vi "EXAMPLE_REQUEST.vi"() -> ()   [LabVIEW 2016]
uses:
  Response/Response.lvclass
panel:
  in  "Request":T1(ring)=enum."PATCH"
  out "Response Headers":string
  out "Status Description":string
  out "Status Code":dbl
  out "Response Body":string
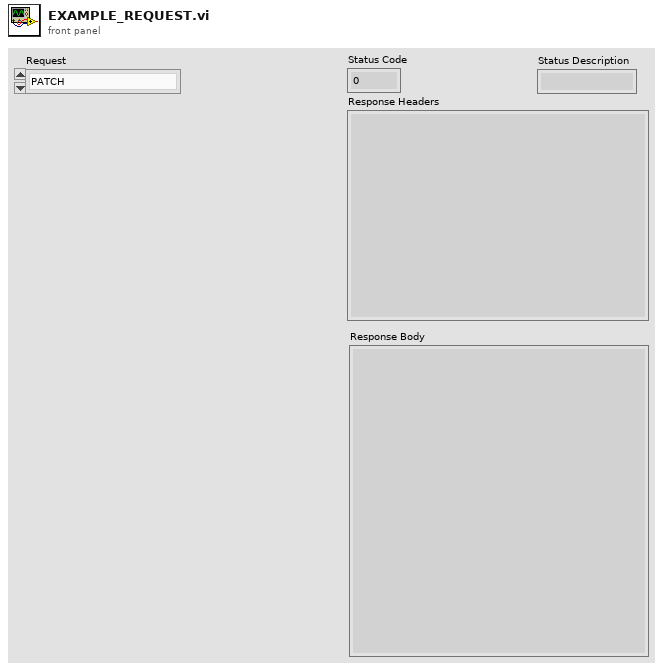
[diagram p1: front panel]
types:
  T1 = enum16{"PATCH_MULTIPART", "POST_MULTIPART", "PATCH", "DELETE", "HEAD", "PUT", "GET"}
  T2 = cluster{"Name":string, "Value":string, "File":path, "Filename":string, "MIME type":string}[]
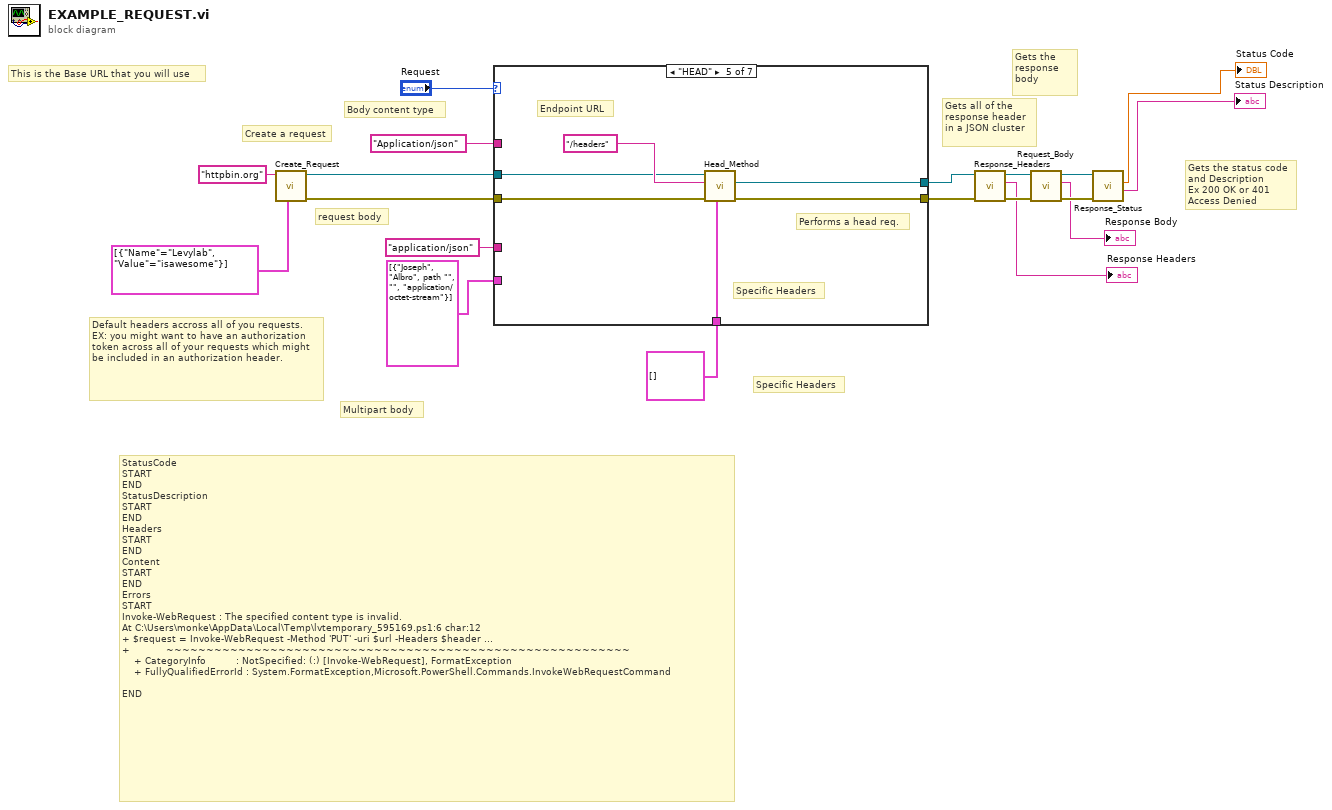
[diagram p0: block diagram]
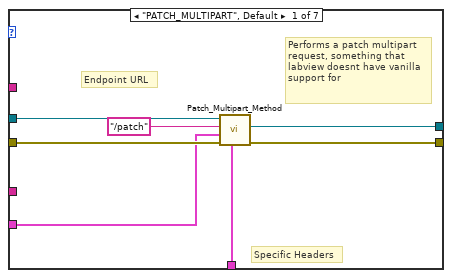
[diagram p2: hidden frame]
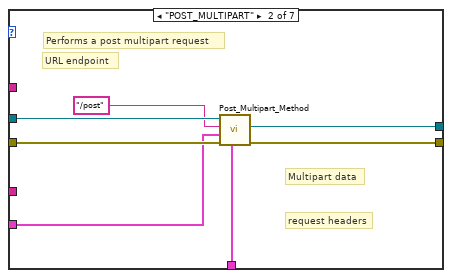
[diagram p3: hidden frame]
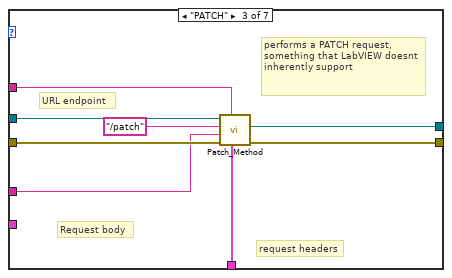
[diagram p4: hidden frame]
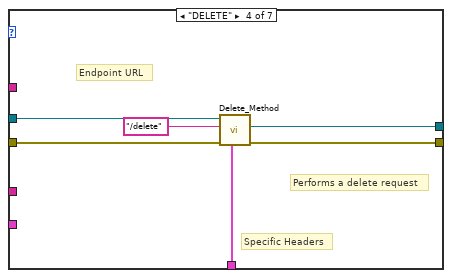
[diagram p5: hidden frame]
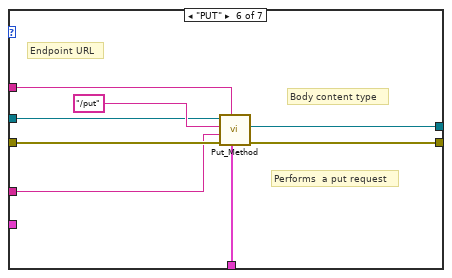
[diagram p6: hidden frame]
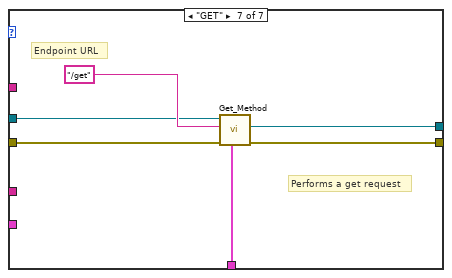
[diagram p7: hidden frame]
diagram:
  # "StatusCode\nSTART\nEND\nStatusDescription\nSTART\nEND\nHeaders\nSTART\nEND\nContent\nSTART\nEND\nErrors\nSTART\nInvoke-WebRequest : The specified content type is invalid.\nAt C:\\Users\\monke\\AppData\\Local\\Temp\\lvtemporary_595169.ps1:6 char:12\n+ $request = Invoke-WebRequest -Method 'PUT' -uri $url -Headers $header ...\n+            ~~~~~~~~~~~~~~~~~~~~~~~~~~~~~~~~~~~~~~~~~~~~~~~~~~~~~~~~~~\n    + CategoryInfo          : NotSpecified: (:) [Invoke-WebRequest], FormatException\n    + FullyQualifiedErrorId : System.FormatException,Microsoft.PowerShell.Commands.InvokeWebRequestCommand\n \nEND"
  # "Multipart body"
  # "request body"
  # "Body content type"
  # "Specific Headers"
  # "Gets the status code and Description\nEx 200 OK or 401 Access Denied"
  # "Gets the response body"
  # "Gets all of the response header in a JSON cluster"
  # "Default headers accross all of you requests.\nEX: you might want to have an authorization token across all of your requests which might be included in an authorization header."
  # "This is the Base URL that you will use"
  # "Create a request"
  n1 = call "Create_Request.vi"("Headers"=cluster{"Name":string, "Value":string}[] [{"Name"="Levylab", "Value"="isawesome"}], "Base URL"="httpbin.org") -> ("error out"=w12:errorcluster, "Request out"=w19:refnum<class "Request.lvclass">)  [unwired: 8 in]
  n2 = case shown="\"HEAD\"" "Request" {
    tunnel: w19 -> [w25 w33 w41 w47 w52 w60 w66]
    tunnel: [w24 w31 w39 w46 w51 w59 w65] -> w15
    tunnel: w12 -> [w23 w30 w38 w45 w50 w58 w64]
    tunnel: [w22 w29 w37 w44 w49 w57 w63] -> w11
    tunnel: cluster{"Name":string, "Value":string}[] [] ("Headers") -> [w21 w28 w36 w42 w48 w56 w62]
    tunnel: T2 [{"Name"="Joseph", "Value"="Albro", "File"=path "", "Filename"="", "MIME type"="application/octet-stream"}] ("Multpart/Form-Data") -> [w20 w27 _ _ _ _ _]
    tunnel: "Application/json" ("Body Content-Type") -> [_ _ w35 _ _ w55 _]
    tunnel: "application/json" ("Body") -> [_ _ w34 _ _ w54 _]
    frame "PATCH_MULTIPART", Default {
      # "Performs a patch multipart request, something that labview doesnt have vanilla support for"
      # "Specific Headers"
      # "Endpoint URL"
      n3 = call "Patch_Multipart_Method.vi"("Headers"=w21, "error in (no error)"=w23, "Multpart/Form-Data"=w20, "Endpoint URL"="/patch", "Request in"=w25) -> ("error out"=w22:errorcluster, "Response out"=w24:refnum<class "Response.lvclass">)  [unwired: 4 in, 1 out]
    }
    frame "POST_MULTIPART" {
      # "request headers"
      # "Multipart data"
      # "URL endpoint"
      # "Performs a post multipart request"
      n4 = call "Post_Multipart_Method.vi"("Headers"=w28, "error in (no error)"=w30, "Multpart/Form-Data"=w27, "Endpoint URL"="/post", "Request in"=w33) -> ("error out"=w29:errorcluster, "Response out"=w31:refnum<class "Response.lvclass">)  [unwired: 4 in, 1 out]
    }
    frame "PATCH" {
      # "performs a PATCH request, something that LabVIEW doesnt inherently support"
      # "URL endpoint"
      # "Request body"
      # "request headers"
      n5 = call "Patch_Method.vi"("Headers"=w36, "Body Content-Type"=w35, "error in (no error)"=w38, "Body"=w34, "Endpoint URL"="/patch", "Request in"=w41) -> ("error out"=w37:errorcluster, "Response out"=w39:refnum<class "Response.lvclass">)  [unwired: 3 in, 1 out]
    }
    frame "DELETE" {
      # "Endpoint URL"
      # "Specific Headers"
      # "Performs a delete request"
      n6 = call "Delete_Method.vi"("Headers"=w42, "error in (no error)"=w45, "Endpoint URL"="/delete", "Request in"=w47) -> ("error out"=w44:errorcluster, "Response out"=w46:refnum<class "Response.lvclass">)  [unwired: 5 in, 1 out]
    }
    frame "HEAD" {
      # "Performs a head req."
      # "Endpoint URL"
      # "Specific Headers"
      n7 = call "Head_Method.vi"("Headers"=w48, "error in (no error)"=w50, "Endpoint URL"="/headers", "Request in"=w52) -> ("error out"=w49:errorcluster, "Response out"=w51:refnum<class "Response.lvclass">)  [unwired: 5 in, 1 out]
    }
    frame "PUT" {
      # "Performs  a put request"
      # "Body content type"
      # "Endpoint URL"
      n8 = call "Put_Method.vi"("Headers"=w56, "Body Content-Type"=w55, "error in (no error)"=w58, "Body"=w54, "Endpoint URL"="/put", "Request in"=w60) -> ("error out"=w57:errorcluster, "Response out"=w59:refnum<class "Response.lvclass">)  [unwired: 3 in, 1 out]
    }
    frame "GET" {
      # "Endpoint URL"
      # "Performs a get request"
      n9 = call "Get_Method.vi"("Headers"=w62, "error in (no error)"=w64, "Endpoint URL"="/get", "Request in"=w66) -> ("error out"=w63:errorcluster, "Response out"=w65:refnum<class "Response.lvclass">)  [unwired: 5 in, 1 out]
    }
  }
  n10 = call "Response_Headers.vi"("error in (no error)"=w11, "Response in"=w15) -> ("error out"=w10:errorcluster, "Response Headers"=→"Response Headers":string, "Response out"=w14:refnum<class "Response.lvclass">)  [unwired: 7 in]
  n11 = call "Request_Body.vi"("error in (no error)"=w10, "Response in"=w14) -> ("error out"=w9:errorcluster, "Response Body"=→"Response Body":string, "Response out"=w13:refnum<class "Response.lvclass">)  [unwired: 7 in]
  n12 = call "Response_Status.vi"("error in (no error)"=w9, "Response in"=w13) -> ("Status Description"=→"Status Description":string, "Status Code"=→"Status Code":dbl)  [unwired: 6 in, 2 out]
